vi "Vector - Strings.vi"(7 "data type of variable":string[](array[string]), 8 "error in":errorcluster, 10 "variable name":string, 11 "pipe in":T1) -> (0 "error out":errorcluster, 2 "value":string[](array[string]), 3 "pipe out":T1)   [LabVIEW 2013, in "GOLPI library.lvlib"]
uses:
  GOLPI library.lvlib
  LV Process.lvlibp/Pipe Handle.ctl
  <vilib>/Utility/error.llb/Error Cluster From Error Code.vi
  <vilib>/ErrorRing/Error Ring.xnode
  LV Process.lvlibp
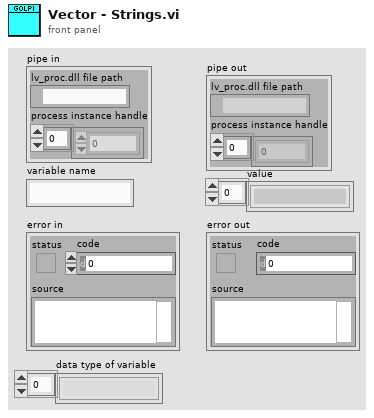
[diagram p1: front panel]
types:
  T1 = typedef "LV Process.lvlibp/Pipe Handle.ctl" = cluster{"lv_proc.dll file path":path, "process instance handle":u32[]}
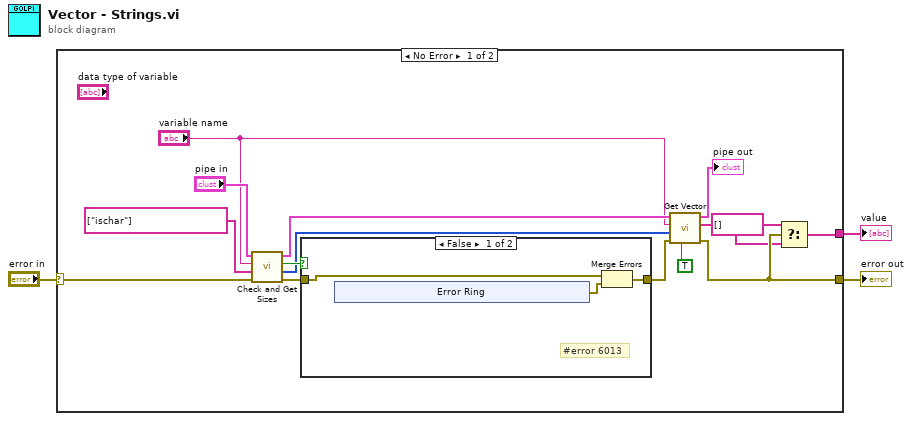
[diagram p0: block diagram]
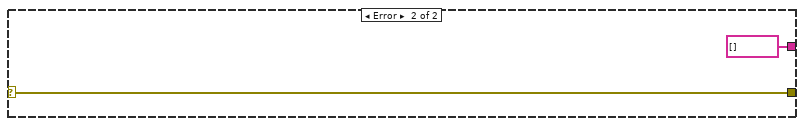
[diagram p3: hidden frame]
diagram:
  n1 = case shown="No Error" "error in" {
    selector: "error in" -> [w15 w29]
    tunnel: [w7 w29] -> w3
    tunnel: [w18 string[] [] ("vector")] -> w1
    frame No Error {
      n2 = call "Check and Get Sizes.vi"("error in (no error)"=w15, "test commands"=string[] ["ischar"], "variable name"="variable name", "pipe in"="pipe in") -> ("error out"=w14:errorcluster, "octave sizes"=w9:i32[], "all tests OK?"=w16:bool, "pipe out"=w12:T1)  [unwired: 4 in]
      n3 = case shown="False" w16 {
        tunnel: w14 -> [w20 w27]
        tunnel: [w19 w27] -> w8
        frame False {
          # "#error 6013"
          n4 = xnode "Error Ring"() -> ("error out"=w21:errorcluster)
          n5 = Merge Errors(w20, w21) -> (w19:errorcluster)
        }
        frame True {
        }
      }
      n6 = call "Get Vector.vi"("no transpose\nfor reading"=TRUE ("no transpose\nwhen reading"), "error in (no error)"=w8, "octave vector sizes"=w9, "variable name"="variable name", "pipe in"=w12) -> ("error out"=w7:errorcluster, "vector"=w6:string[], "pipe out"=→"pipe out":T1)  [unwired: 4 in]
      n7 = Select(t=string[] [], s=w7, f=w6) -> (s? t:f=w18:string[])
    }
    frame Error {
    }
  }
  "value" <- w1
  "error out" <- w3
